vi "Read configuration.vi"(7 "force loading?":bool=TRUE, 8 "error in (no error)":errorcluster, 11 "Template in":refnum<class "BMC.lvclass">) -> (0 "error out":errorcluster, 3 "Template out":refnum<class "BMC.lvclass">)   [LabVIEW 2012, in "BMC.lvclass"]
doc: "Reads the XML-based configuration file and populates the configuration cluster accordingly. Configuration file name is <component ID>.xml."
uses:
  BMC.lvclass
  <vilib>/Distrio/Murmex/Murmex/Murmex.lvclass
  BMC.lvclass/BMC.ctl
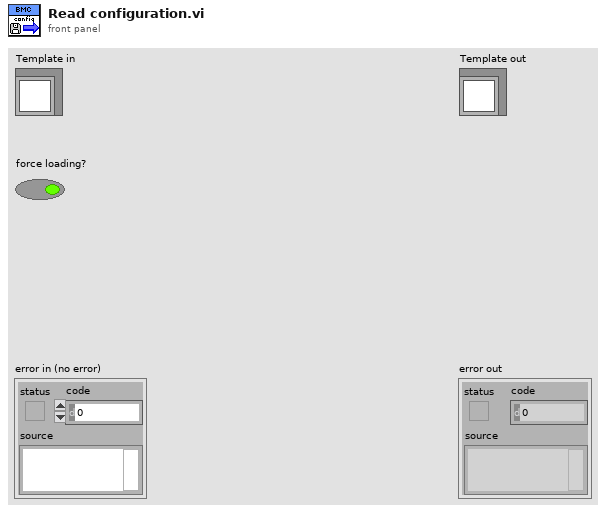
[diagram p1: front panel]
types:
  T1 = typedef "BMC.lvclass/configuration_cluster.ctl" = cluster{"Mapping file":path, "Flat mirror file":path}
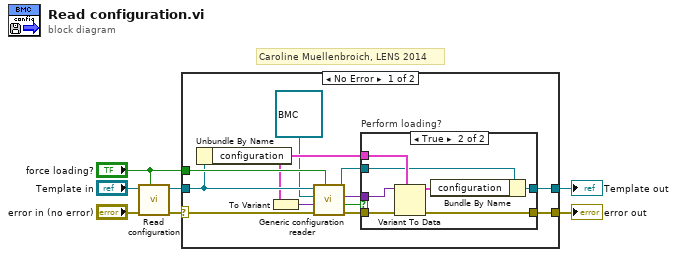
[diagram p0: block diagram]
diagram:
  # "Caroline Muellenbroich, LENS 2014"
  n1 = call-parent "Read configuration.vi"("force loading?"="force loading?", "error in (no error)"="error in (no error)", "Murmex in"="Template in") -> ("error out"=w5:errorcluster, "Murmex out"=w4:refnum<class "BMC.lvclass">)  [unwired: 7 in]
  n2 = case shown="No Error" w5 {
    selector: w5 -> [w16 w30]
    tunnel: [w18 w30] -> w3
    tunnel: [w19 w29] -> w2
    tunnel: w4 -> [w13 w29]
    tunnel: "force loading?" -> [w17 _]
    frame No Error {
      n3 = Unbundle By Name(w13) -> ("configuration"=w11:T1)
      n4 = To Variant(anything=w11) -> (Variant=w12:variant)
      n5 = call <vilib>:"Generic configuration reader.vi"("force loading?"=w17, "error in (no error)"=w16, "configuration cluster variant"=w12, "inheritance level"=refnum<class "BMC.lvclass"> refnum ("Template.lvclass"), "Murmex in"=w13) -> ("error out"=w15:errorcluster, "loaded?"=w9:bool, "configuration data (variant)"=w10:variant, "Murmex out"=w14:refnum<class "BMC.lvclass">)  [unwired: 3 in]
      n6 = case "Perform loading?" shown="True" w9 {
        tunnel: [w21 w22] -> w19
        tunnel: w11 -> [_ w28]
        tunnel: [w20 w27] -> w18
        tunnel: w15 -> [w20 w24]
        tunnel: w14 -> [w21 w26]
        tunnel: w10 -> [_ w23]
        frame False {
        }
        frame True {
          n7 = Variant To Data(error in=w24, type=w28, Variant=w23) -> (data=w25:T1, error out=w27:errorcluster)
          n8 = Bundle By Name(cluster=w26, "configuration"=w25) -> (w22:refnum<class "BMC.lvclass">)
        }
      }
    }
    frame Error {
    }
  }
  "error out" <- w3
  "Template out" <- w2
